vi "Read Power.vi"(0 "SG Path Power Meter Accessor in":refnum<class "SG Path Accessor.lvclass">, 5 "Cal point in":T1, 11 "error in":errorcluster) -> (4 "SG Path Power Meter Accessor out":refnum<class "SG Path Accessor.lvclass">, 6 "Power (dBm)":dbl, 15 "error out":errorcluster)   [LabVIEW 2023, in "RS NRPx Power Meter.lvlib" / "SG Path Accessor.lvclass"]
uses:
  SG Path Accessor.lvclass
  Public/Base Classes/Scalar/Scalar Path/Type Definitions/Cal Point.ctl
  Power Meter/Power Meter.lvclass
  Power Meter/Power Meter.lvclass/Power Meter.ctl
  Power Meter/Properties/Read Resource Name.vi
  Instruments/Power Meter/Power Meter Factory/Power Meter Factory.lvclass
  <instrlib>/Rohde&Schwarz Power Meter/Rohde&Schwarz Power Meter.lvlib
  Public/Base Classes/Scalar/Scalar Path/Scalar Path.lvclass
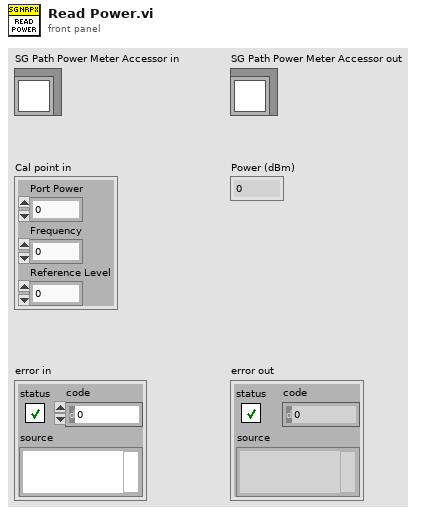
[diagram p1: front panel]
types:
  T1 = typedef "RFFixtureCharact.Public.lvlib/Scalar Path.lvclass/Cal Point.ctl" = cluster{"Port Power":dbl, "Frequency":dbl, "Reference Level":dbl}
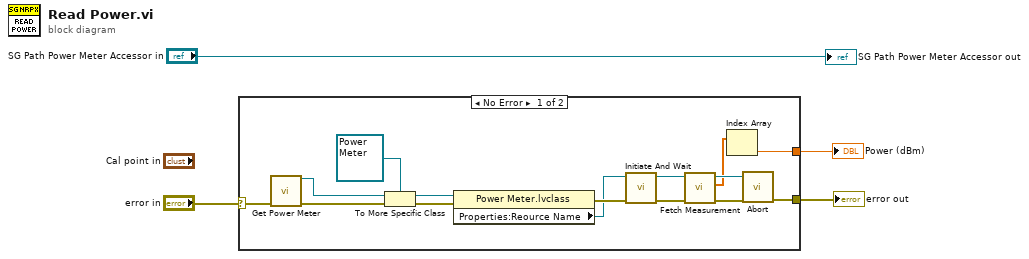
[diagram p0: block diagram]
diagram:
  n1 = case shown="No Error" "error in" {
    selector: "error in" -> [w19 w20]
    tunnel: [w11 w20] -> w3
    tunnel: [w5 _] -> w1
    frame No Error {
      n2 = call "Get Power Meter.vi"("error in (no error)"=w19) -> ("Power Meter Base out"=w15:refnum<class "Power Meter Base.lvclass">, "error out"=w14:errorcluster)  [unwired: 13 in]
      n3 = To More Specific Class(target class=refnum<class "Power Meter.lvclass"> refnum ("PM NI568X in"), reference=w15, error in=w14) -> (specific class reference=w17:refnum<class "Power Meter.lvclass">, error out=w18:errorcluster)
      n4 = property class="Power Meter.lvclass"(reference=w17, error in=w18) -> (error out=w10:errorcluster, "Properties:Reource Name"=w7:refnum<visa-resource-name>)  [unwired: 1 out]
      n5 = call <instrlib>:"Initiate And Wait.vi"("error in (no error)"=w10, "VISA resource name"=w7) -> ("error out"=w9:errorcluster, "VISA resource name out"=w8:refnum<visa-resource-name>)  [unwired: 8 in]
      n6 = call <instrlib>:"Fetch Measurement.vi"("error in (no error)"=w9, "VISA resource name"=w8) -> ("error out"=w12:errorcluster, "Measurement"=w6:dbl[], "VISA resource name out"=w13:refnum<visa-resource-name>)  [unwired: 7 in]
      n7 = Index Array(array=w6) -> (element=w5:dbl)  [unwired: 1 in]
      n8 = call <instrlib>:"Abort.vi"("error in (no error)"=w12, "VISA resource name"=w13) -> ("error out"=w11:errorcluster)  [unwired: 8 in, 1 out]
    }
    frame Error {
    }
  }
  "error out" <- w3
  "Power (dBm)" <- w1
  "SG Path Power Meter Accessor out" <- "SG Path Power Meter Accessor in"
